vi "Place Pick up tool on baseplate.vi"   [LabVIEW 2020]
uses:
  Classes/Workspace/Pick Up Tool Area/Pick Up Tool Fixture.lvclass
  Classes/Workspace/Carrier Tray/Assembly Tray.lvclass
  Classes/Routine/Pick and Place/Pick and Place Type.ctl
  Classes/Routine/Pick and Place/Pick and Place.lvclass
  Classes/Routine/Pick and Place/Pick and Place.lvclass/Pick and Place.ctl
  Classes/Routine/Pick and Place/Write Pick and Place Type.vi
  Classes/Controller/Controller.lvclass
  Classes/Controller/I-O/I-O.lvclass
  Classes/Controller/Dispenser/Dispenser.lvclass
types:
  T1 = typedef "Pick and Place.lvclass/Pick and Place Type.ctl" = enum16{"Primary Pick Up", "Secondary Pick Up", "Put Down All", "Pick Up All", "Put Down Secondary"}
  T2 = typedef "Controller.lvclass/Controllers.ctl" = cluster{"I-O.lvclass":refnum<class "I-O.lvclass">, "Dispenser.lvclass":refnum<class "Dispenser.lvclass">, "Gantry":refnum<k24>}
  T3 = typedef "Fixture.lvclass/Workspace.ctl" = cluster{"XYZTheta":dbl[], "Workspace Valve":i32, "Workspace Sensor":i32}
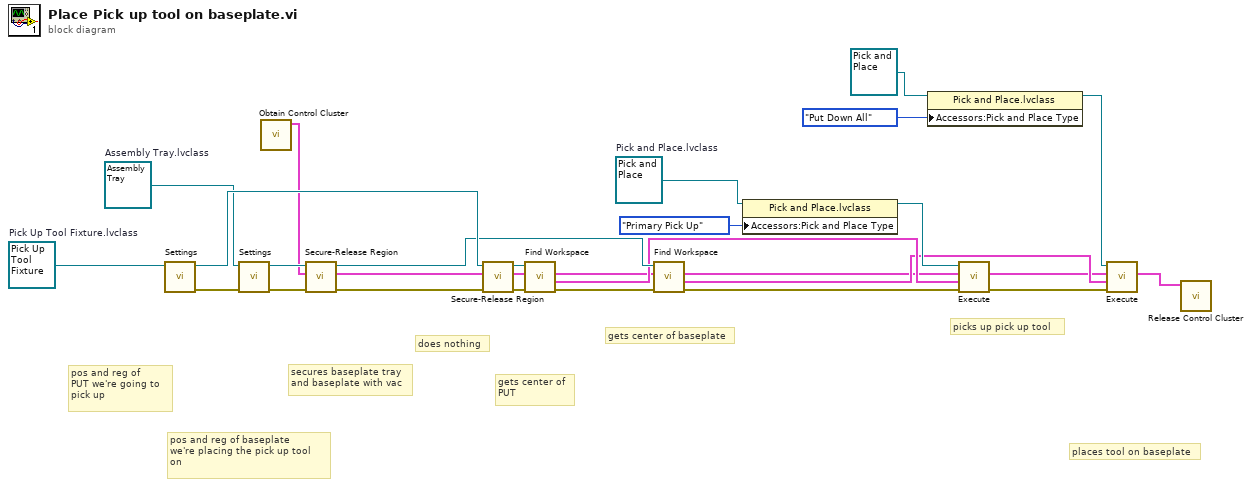
[diagram p0: block diagram]
diagram:
  w17 = refnum<class "Pick and Place.lvclass"> refnum  # Pick and Place.lvclass
  w24 = refnum<class "Assembly Tray.lvclass"> refnum  # Assembly Tray.lvclass
  w28 = refnum<class "Pick Up Tool Fixture.lvclass"> refnum  # Pick Up Tool Fixture.lvclass
  # "places tool on baseplate"
  # "picks up pick up tool"
  # "gets center of baseplate"
  # "gets center of \nPUT"
  # "does nothing"
  # "secures baseplate tray\nand baseplate with vac"
  # "pos and reg of baseplate\nwe're placing the pick up tool \non"
  # "pos and reg of\nPUT we're going to\npick up"
  n1 = call-dynamic "Settings.vi"("Workspace in"=w28) -> ("error out"=w21:errorcluster, "Workspace out"=w27:refnum<class "Pick Up Tool Fixture.lvclass">)  [unwired: 9 in]
  n2 = call-dynamic "Settings.vi"("error in (no error)"=w21, "Assembly Tray In"=w24) -> ("error out"=w20:errorcluster, "Assembly Tray Out"=w23:refnum<class "Assembly Tray.lvclass">)  [unwired: 8 in]
  n3 = call "Obtain Control Cluster.vi"() -> ("Control Out"=w2:T2)  [unwired: 11 in]
  n4 = call-dynamic "Secure-Release Region.vi"("error in (no error)"=w20, "Control In"=w2, "Carrier Tray in"=w23) -> ("error out"=w19:errorcluster, "Control Out"=w1:T2, "Carrier Tray out"=w22:refnum<class "Assembly Tray.lvclass">)  [unwired: 6 in]
  n5 = call-dynamic "Secure-Release Region.vi"("error in (no error)"=w19, "Control In"=w1, "Fixture in"=w27) -> ("error out"=w25:errorcluster, "Control Out"=w7:T2, "Fixture out"=w26:refnum<class "Pick Up Tool Fixture.lvclass">)  [unwired: 6 in]
  n6 = call-dynamic "Find Workspace.vi"("Error In"=w25, "Control In"=w7, "Workspace In"=w26) -> ("Error Out"=w18:errorcluster, "Workspace Out"=w14:T3, "Control Out"=w6:T2)  [unwired: 5 in, 1 out]
  n7 = call-dynamic "Find Workspace.vi"("Error In"=w18, "Control In"=w6, "Carrier Tray in"=w22) -> ("Error Out"=w13:errorcluster, "Workspace"=w5:T3, "Control Out"=w4:T2)  [unwired: 5 in, 1 out]
  n8 = property class="Pick and Place.lvclass"(reference=w17, "Accessors:Pick and Place Type"=Pick_and_Place_Type."Primary Pick Up" ("Pick and Place Type")) -> (reference out=w15:refnum<class "Pick and Place.lvclass">)  [unwired: 1 in, 1 out]
  n9 = property class="Pick and Place.lvclass"(reference=refnum<class "Pick and Place.lvclass"> refnum ("Pick and Place.lvclass"), "Accessors:Pick and Place Type"=Pick_and_Place_Type."Put Down All" ("Pick and Place Type")) -> (reference out=w9:refnum<class "Pick and Place.lvclass">)  [unwired: 1 in, 1 out]
  n10 = call-dynamic "Execute.vi"("error in (no error)"=w13, "Workspace"=w14, "Cluster"=w4, "Pick and Place in"=w15) -> ("error out"=w10:errorcluster, "Control Out"=w3:T2)  [unwired: 5 in, 1 out]
  n11 = call-dynamic "Execute.vi"("error in (no error)"=w10, "Workspace"=w5, "Cluster"=w3, "Pick and Place in"=w9) -> ("Control Out"=w8:T2)  [unwired: 5 in, 2 out]
  n12 = call "Release Control Cluster.vi"("output cluster"=w8) -> ()  [unwired: 11 in]
